vi "PenaltyDefenseSkill.vi"(4 "Game in":refnum<class "Game.lvclass">, 6 "PenaltyOurKick?":bool, 8 "error in (no error)":errorcluster, 9 "IndexInVector":dbl, 10 "Robot":refnum<class "Robot.lvclass">, 11 "PenaltyDefenseSkill in":refnum<class "PenaltyDefenseSkill.lvclass">) -> (0 "error out":errorcluster, 2 "Robot out":refnum<class "Robot.lvclass">, 3 "PenaltyDefenseSkill out":refnum<class "PenaltyDefenseSkill.lvclass">)   [LabVIEW 2020, in "PenaltyDefenseSkill.lvclass"]
uses:
  PenaltyDefenseSkill.lvclass
  Robot_class/Robot.lvclass
  Game_class/Game.lvclass
  Game_class/Game.lvclass/Game.ctl
  Robot_class/Robot.lvclass/Robot.ctl
  Game_class/Read FieldRef.vi
  Game_class/Read NewParameters.vi
  Robot_class/Write dest_x.vi
  Robot_class/Write dest_y.vi
  Robot_class/Write dest_orientation.vi
  Field_class/Field.lvclass
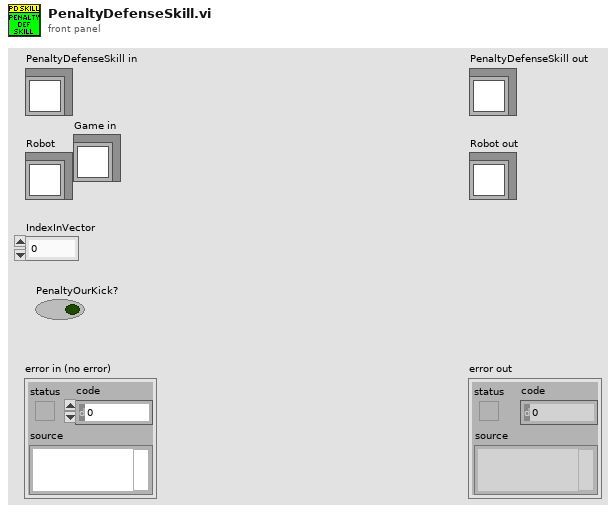
[diagram p1: front panel]
types:
  T1 = typedef "NewParameters.ctl" = cluster{"PenaltyDistance":dbl, "DistanceAttackerToBackBall":dbl, "Division":enum16{"Div B", "Div A"}, "DistanceToAvoidyEnemyRobot":dbl, "BallPlacementDistance":dbl, "DisatanceBehindBallToStealBall":dbl}
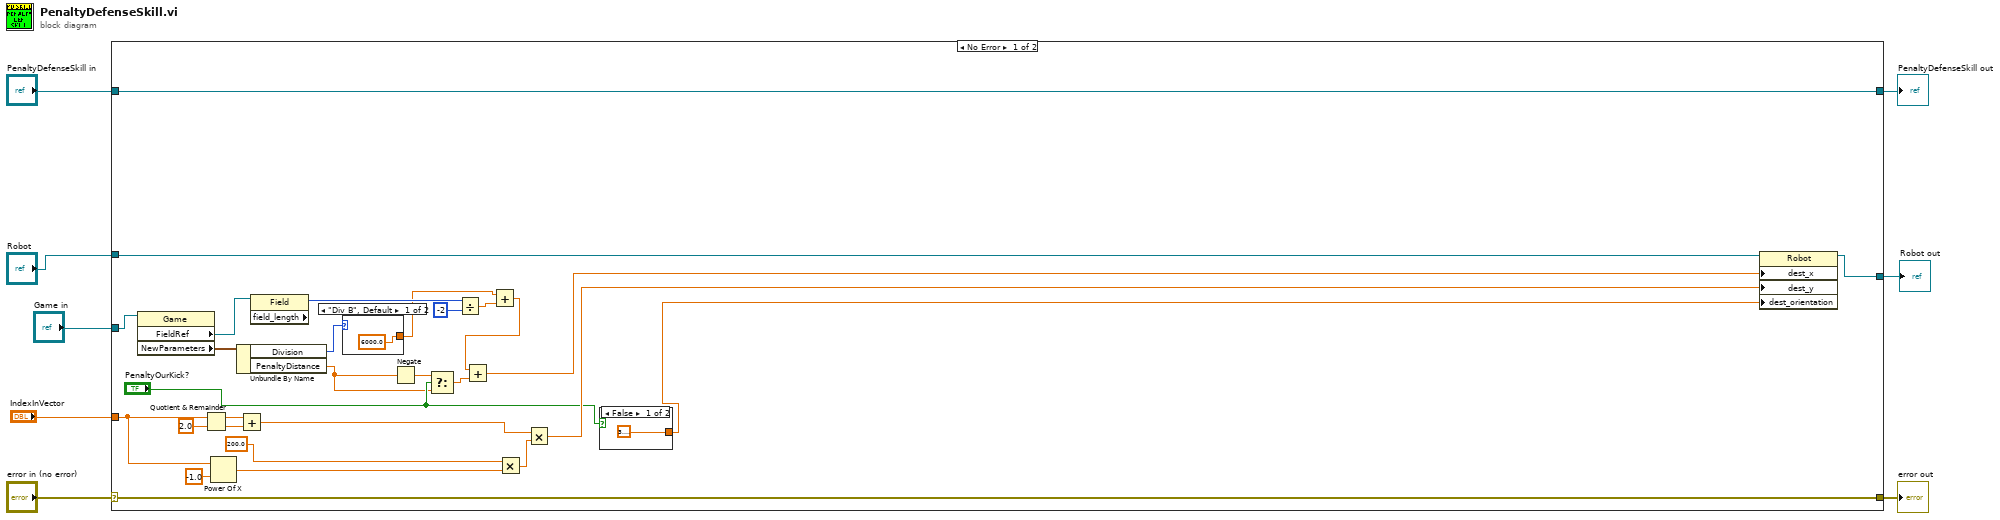
[diagram p0: block diagram]
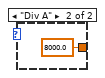
[diagram p2: hidden frame]
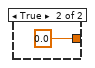
[diagram p3: hidden frame]
diagram:
  n1 = case shown="No Error" "error in (no error)" {
    selector: "error in (no error)" -> [w36 w44]
    tunnel: [w36 w44] -> w7
    tunnel: [w37 w43] -> w5
    tunnel: "PenaltyDefenseSkill in" -> [w37 w43]
    tunnel: "IndexInVector" -> [w32 _]
    tunnel: "Robot" -> [w26 w42]
    tunnel: [w23 w42] -> w2
    tunnel: "Game in" -> [w22 _]
    frame No Error {
      n2 = property class="Game"(reference=w22) -> ("FieldRef"=w15:refnum<class "Field.lvclass">, "NewParameters"=w17:T1)  [unwired: 1 in, 2 out]
      n3 = Quotient & Remainder(x=w32, y=2.0) -> (x-y*floor(x/y)=w34:dbl, floor(x/y)=w33:dbl)
      n4 = Power Of X(1:-1.0 ("x"), 2:w32) -> (0:w30:dbl)
      n5 = Unbundle By Name(w17) -> ("Division"=w11:enum16{"Div B", "Div A"}, "PenaltyDistance"=w16:dbl)
      n6 = Add(x=w34, y=w33) -> (x+y=w28:dbl)
      n7 = property class="Field"(reference=w15) -> ("field_length"=w14:i32)  [unwired: 1 in, 2 out]
      n8 = case shown="\"Div B\", Default" w11 {
        tunnel: [6000.0 8000.0] -> w10
        frame "Div B", Default {
        }
        frame "Div A" {
        }
      }
      n9 = Negate(x=w16) -> (-x=w20:dbl)
      n10 = Select(t=w20, s="PenaltyOurKick?", f=w16) -> (s? t:f=w19:dbl)
      n11 = Divide(x=w14, y=-2) -> (x/y=w12:dbl)
      n12 = Add(x=w10, y=w12) -> (x+y=w9:dbl)
      n13 = Add(x=w9, y=w19) -> (x+y=w18:dbl)
      n14 = Multiply(x=200.0, y=w30) -> (x*y=w27:dbl)
      n15 = Multiply(x=w28, y=w27) -> (x*y=w25:dbl)
      n16 = case shown="False" "PenaltyOurKick?" {
        tunnel: [3.141592653589793 0.0 ("x")] -> w24
        frame False {
        }
        frame True {
        }
      }
      n17 = property class="Robot"(reference=w26, "dest_x"=w18, "dest_y"=w25, "dest_orientation"=w24) -> (reference out=w23:refnum<class "Robot.lvclass">)  [unwired: 1 in, 1 out]
    }
    frame Error {
    }
  }
  "error out" <- w7
  "PenaltyDefenseSkill out" <- w5
  "Robot out" <- w2
